vi "MatchRegExResultOnly.vi"(5 "capture index":i32, 7 "Options":cluster{"Create":u32, "Match":u32} {"Match" format="%.0x"; "Create" format="%.0x"}, 8 "error in":errorcluster, 9 "offset (0)":i32, 10 "search pattern":string, 11 "string":string) -> (0 "error out":errorcluster, 1 "NoMatch?":bool)   [LabVIEW 2021]
uses:
  Pcre2GetOvectorPointer8.vi
  Pcre2MoOfSubstrNumFmOv.vi
  Pcre2CompileError.vi
  Pcre2ErrorNull.vi
  Pcre2LibError.vi
  Pcre2FnkCallError.vi
  libpcre2-8.lvlib
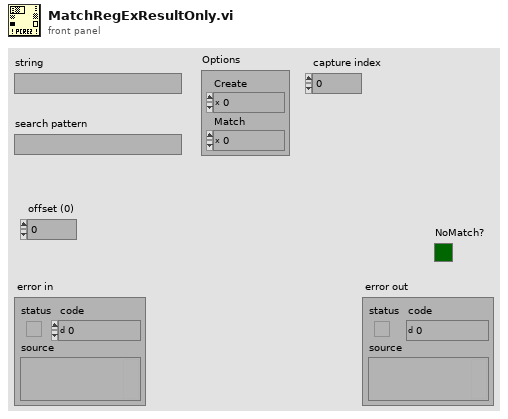
[diagram p1: front panel]
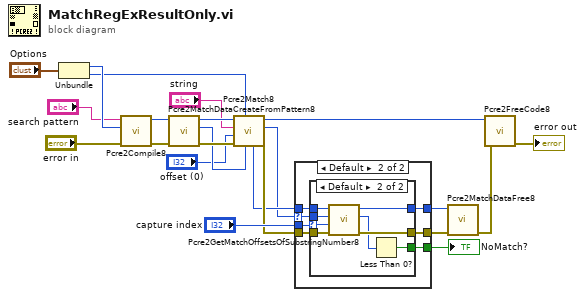
[diagram p0: block diagram]
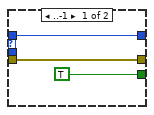
[diagram p2: hidden frame]
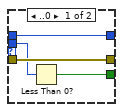
[diagram p3: hidden frame]
diagram:
  n1 = Unbundle("Options") -> ("Create"=w13:u32, "Match"=w12:u32)
  n2 = call "Pcre2Compile8.vi"("error in"="error in", "Options"=w13, "Pattern"="search pattern") -> ("error out"=w19:errorcluster, "pCode"=w18:u64)  [unwired: 7 in]
  n3 = call "Pcre2MatchDataCreateFromPattern8.vi"("error in"=w19, "pCode"=w18) -> ("error out"=w20:errorcluster, "pMatchData"=w7:u64, "pCode"=w21:u64)  [unwired: 7 in]
  n4 = call "Pcre2Match8.vi"("pMatchData"=w7, "Options"=w12, "error in"=w20, "StartOffset"="offset (0)", "Subject"="string", "pCode"=w21) -> ("error out"=w11:errorcluster, "MatchResult"=w1:i32, "pCode"=w17:u64, "pMatchData"=w8:u64)  [unwired: 2 in]
  n5 = case shown="Default" w1 {
    selector: w1 -> [_ w27]
    tunnel: "capture index" -> [_ w26]
    tunnel: w11 -> [w24 w32]
    tunnel: [w25 w31] -> w10
    tunnel: [w24 w30] -> w9
    tunnel: w8 -> [w25 w29]
    tunnel: [TRUE w28] -> w2
    frame ..-1 {
    }
    frame Default {
      n6 = case shown="Default" w26 {
        selector: w26 -> [_ w37]
        tunnel: w32 -> [w35 w44]
        tunnel: [w36 w43] -> w31
        tunnel: [w35 w42] -> w30
        tunnel: w29 -> [w36 w41]
        tunnel: [w33 w40] -> w28
        tunnel: w27 -> [w34 w38]
        frame ..0 {
          n7 = Less Than 0?(x=w34) -> (x < 0?=w33:bool)
        }
        frame Default {
          n8 = call "Pcre2GetMatchOffsetsOfSubstringNumber8.vi"("error in"=w44, "Number"=w37, "MatchResult"=w38, "pMatchData"=w41) -> ("error out"=w42:errorcluster, "MatchOffset"=w39:i32, "pMatchData"=w43:u64)  [unwired: 4 in, 1 out]
          n9 = Less Than 0?(x=w39) -> (x < 0?=w40:bool)
        }
      }
    }
  }
  "NoMatch?" <- w2
  n10 = call "Pcre2MatchDataFree8.vi"("error in"=w9, "pMatchData"=w10) -> ("error out"=w16:errorcluster)  [unwired: 9 in]
  n11 = call "Pcre2FreeCode8.vi"("error in"=w16, "pCode"=w17) -> ("error out"=→"error out":errorcluster)  [unwired: 9 in]
